vi "rqcBob Picture Demo (Low Level Example).vi"() -> ()   [LabVIEW 2019]
panel:
  in  "Corrected Bob's key":path
  in  "Alices's port":string
  in  "Alices's IP":string
  out "pyton script path":path=path "../python_scripts/cascade_alice.py"
  in  "error in":errorcluster
  out "?":picture
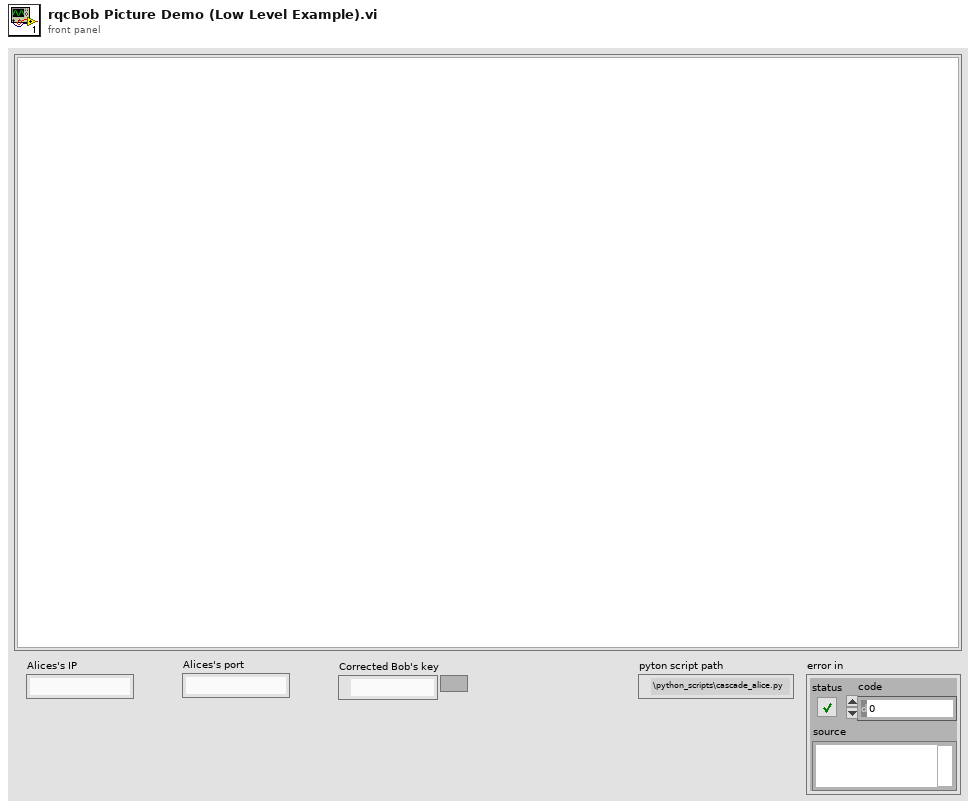
[diagram p1: front panel]
types:
  T1 = typedef "imagedata.ctl" = cluster{"image type":i32, "image depth":i32, "image":u8[], "mask":u8[], "colors":u32[], "Rectangle":cluster{"left":i16, "top":i16, "right":i16, "bottom":i16}}
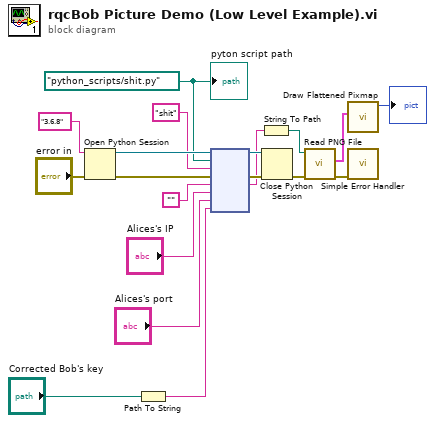
[diagram p0: block diagram]
diagram:
  w12 = path "python_scripts/shit.py" ("module path")
  n1 = Open Python Session(python version="3.6.8" ("Python version"), 3:"error in") -> (session out=w16:refnum<k35>, error out=w15:errorcluster)  [unwired: 1 in]
  n2 = Path To String(path="Corrected Bob's key") -> (string=w2:string)
  n3 = node(w16, w12, "shit" ("function name"), w15, "", "Alices's IP", "Alices's port", w2) -> (w14:refnum<k35>, w8:errorcluster, w7:string)  [unwired: 3 in, 2 out]
  n4 = String To Path(string=w7) -> (path=w6:path)
  n5 = Close Python Session(session in=w14, error in=w8) -> (11:w4:errorcluster)
  n6 = call <vilib>:"Read PNG File.vi"("error in (no error)"=w4, "path to PNG file"=w6) -> ("error out"=w3:errorcluster, "image data"=w19:T1)  [unwired: 7 in, 1 out]
  n7 = call <vilib>:"Draw Flattened Pixmap.vi"("image data"=w19) -> ("new picture"=→"?":picture)  [unwired: 8 in]
  n8 = call <vilib>:"Simple Error Handler.vi"("error in (no error)"=w3) -> ()  [unwired: 4 in, 5 out]
  "pyton script path" <- w12
